vi "Bit depth autoranger.vi"(3 "Scan rate (mV/s)":dbl) -> (0 "I bit depth setting":u8, 1 "V bit depth setting":u8)   [LabVIEW 2015]
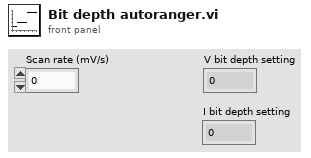
[diagram p1: front panel]
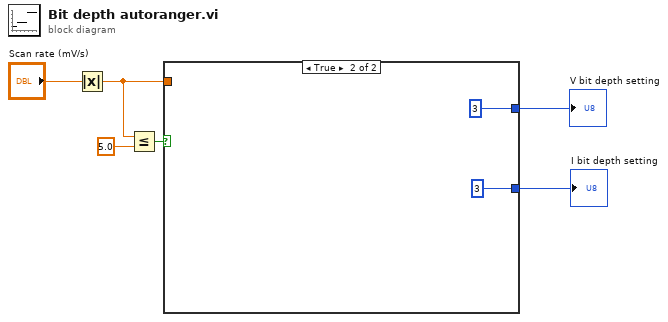
[diagram p0: block diagram]
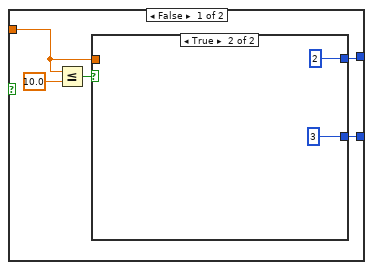
[diagram p2: hidden frame]
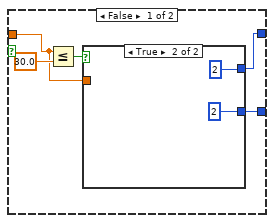
[diagram p3: hidden frame]
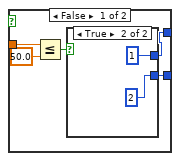
[diagram p4: hidden frame]
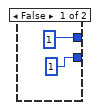
[diagram p5: hidden frame]
diagram:
  n1 = Absolute Value(x="Scan rate (mV/s)") -> (abs(x)=w3:dbl)
  n2 = Less Or Equal?(x=w3, y=5.0) -> (x <= y?=w6:bool)
  n3 = case shown="True" w6 {
    tunnel: w3 -> [w8 _]
    tunnel: [w9 u8 3] -> w4
    tunnel: [w7 u8 3] -> w1
    frame False {
      n4 = Less Or Equal?(x=w8, y=10.0) -> (x <= y?=w10:bool)
      n5 = case shown="True" w10 {
        tunnel: [w14 u8 2] -> w9
        tunnel: w8 -> [w12 _]
        tunnel: [w13 u8 3] -> w7
        frame False {
          n6 = Less Or Equal?(x=w12, y=30.0) -> (x <= y?=w15:bool)
          n7 = case shown="True" w15 {
            tunnel: [w18 u8 2] -> w14
            tunnel: [w17 u8 2] -> w13
            tunnel: w12 -> [w20 _]
            frame False {
              n8 = Less Or Equal?(x=w20, y=50.0) -> (x <= y?=w19:bool)
              n9 = case shown="True" w19 {
                tunnel: [u8 1 u8 1] -> w18
                tunnel: [u8 1 u8 2] -> w17
                frame False {
                }
                frame True {
                }
              }
            }
            frame True {
            }
          }
        }
        frame True {
        }
      }
    }
    frame True {
    }
  }
  "V bit depth setting" <- w4
  "I bit depth setting" <- w1
